vi "Translate Data.vi"(8 "error in (no error)":errorcluster, 10 "DataBuffer":string, 11 "Alicat Controller in":refnum<class "Alicat Controller.lvclass">) -> (0 "error out":errorcluster, 2 "Data":refnum<class "Data.lvclass">, 3 "Alicat Controller out":refnum<class "Alicat Controller.lvclass">)   [LabVIEW 2015, in "Alicat.lvlib" / "Alicat Controller.lvclass"]
doc: "VI used to translate the data buffer to something meaningful (implementation dependent). This VI must be overridden."
uses:
  Alicat Controller.lvclass
  Reusable/Data/Data.lvclass
  Alicat.lvclass
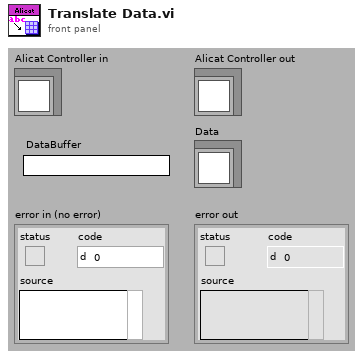
[diagram p1: front panel]
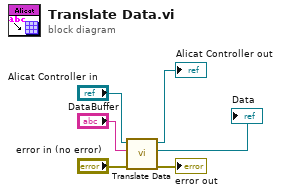
[diagram p0: block diagram]
diagram:
  n1 = call-parent "Translate Data.vi"("error in (no error)"="error in (no error)", "BufferIn"="DataBuffer", "Alicat in"="Alicat Controller in") -> ("error out"=→"error out":errorcluster, "DataOut"=→"Data":refnum<class "Data.lvclass">, "Alicat out"=→"Alicat Controller out":refnum<class "Alicat Controller.lvclass">)  [unwired: 6 in]
